vi "Scratchpad.vi"() -> ()   [LabVIEW 2020]
uses:
  TSnax/Engine/Engine.lvclass
  TSnax/SequenceFile/SequenceFile.lvclass
  TSnax/TS License Type.ctl
  TSnax/TSnax.lvlib
panel:
  out "error out":errorcluster
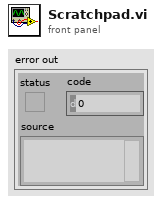
[diagram p1: front panel]
types:
  T1 = typedef "TSnax.lvlib/TS License Type.ctl" = enum16{"Operator", "CustomEditor", "SequenceEditor"}
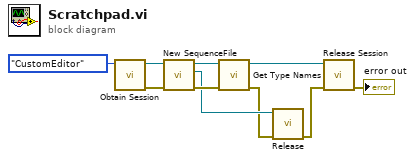
[diagram p0: block diagram]
diagram:
  n1 = call "Obtain Session.vi"("TS License Type (Operator)"=TS_License_Type."CustomEditor") -> ("error out"=w8:errorcluster, "Engine out"=w7:refnum<class "Engine.lvclass">)  [unwired: 9 in]
  n2 = call "New SequenceFile.vi"("error in (no error)"=w8, "Engine in"=w7) -> ("error out"=w5:errorcluster, "New SequenceFile"=w4:refnum<class "SequenceFile.lvclass">, "Engine out"=w6:refnum<class "Engine.lvclass">)  [unwired: 7 in]
  n3 = call "Get Type Names.vi"("error in (no error)"=w5, "Engine in"=w6) -> ("error out"=w3:errorcluster, "Engine out"=w10:refnum<class "Engine.lvclass">)  [unwired: 8 in]
  n4 = call-dynamic "Release.vi"("error in (no error)"=w3, "SequenceFile in"=w4) -> ("error out"=w2:errorcluster)  [unwired: 9 in]
  n5 = call "Release Session.vi"("error in (no error)"=w2, "Engine in"=w10) -> ("error out"=→"error out":errorcluster)  [unwired: 9 in]
